vi "Main.vi"() -> ()   [LabVIEW 2015, in "ROOT.lvlib"]
doc: "This template is based off of the Queued Message Handler design pattern and the Queued Message Handler project template that ships with LabVIEW.\n\nThe main difference is that the queue is private to this module and communication between modules is performed via Broadcast and Request events.\n\nRequest events are wrapped in public API methods and are handled in the Event Handling Loop (EHL) of this VI. Any module can register for Broadcast events sent by this module. The EHL generates messages based on user interface actions.\n\nThe Message Handling Loop (MHL) processes messages generated by the EHL, or by other messages. The messages are string values, so new messages can be added easily to the Message Cases case structure in the MHL. Each message cluster can also provide an optional value for Message Data, which is a variant that can be converted to whatever message-specific data is required.\n_____\nBased on Delacor QMH Project Template 4.2.1.64."
uses:
  ROOT.lvlib
  <vilib>/Delacor/Delacor QMH/Libraries/Module Admin_class/Delacor_lib_QMH_Module Admin.lvclass
  Module Data--cluster.ctl
  <vilib>/Delacor/Delacor QMH/Libraries/Message Queue_class/Delacor_lib_QMH_Message Queue.lvclass/Delacor_lib_QMH_Message Queue.ctl
  Stop Argument--cluster.ctl
  <vilib>/Delacor/Delacor QMH/Libraries/Module Admin_class/Delacor_lib_QMH_Module Admin.lvclass/Delacor_lib_QMH_Module Admin.ctl
  <vilib>/Utility/miscctls.llb/LVPointTypeDef.ctl
  <vilib>/Delacor/Delacor QMH/Libraries/Message Queue_class/Delacor_lib_QMH_Enqueue Message (Single).vi
  <vilib>/Delacor/Delacor QMH/Libraries/Module Admin_class/Delacor_lib_QMH_Get External Launch.vi
  <vilib>/Utility/error.llb/Error Cluster From Error Code.vi
  <vilib>/ErrorRing/Error Ring.xnode
  <vilib>/Delacor/Delacor QMH/Libraries/Message Queue_class/Delacor_lib_QMH_Message Queue.lvclass
  Control/Control.lvlib
panel:
  in  "Stop Thermo Chamber":bool
  out "Initialized?":bool
  in  "Starting Temperature":dbl format="%#_13g"
  in  "Start Thermochamber":bool
  out "Hardware Alias":string
  in  "Get Hardware Number":bool
  in  "Simulate MHL Error":bool
  in  "Simulate EHL Error":bool
  out "error out":errorcluster
  in  "Module Admin":refnum<class "Delacor_lib_QMH_Module Admin.lvclass">
  out "Status":string
  # "ROOT Module\n**This module could be used to launch lots of other hardware modules and used to link them to the rest of the application**"
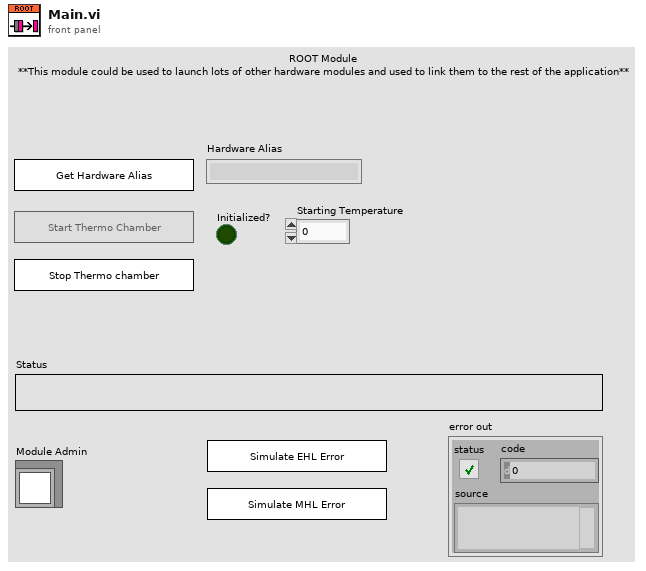
[diagram p1: front panel]
types:
  T1 = typedef "ROOT.lvlib/Request Events--cluster.ctl" = cluster{"Stop Module":refnum<user-event>, "Show Panel":refnum<user-event>, "Hide Panel":refnum<user-event>, "Get Module Execution Status":refnum<user-event>, "Show Diagram":refnum<user-event>}
  T2 = typedef "Control.lvlib/Broadcast Events--cluster.ctl" = cluster{"Module Did Init":refnum<user-event>, "Status Updated":refnum<user-event>, "Error Reported":refnum<user-event>, "Module Did Stop":refnum<user-event>, "Update Module Execution Status":refnum<user-event>, "Thermochamber Started":refnum<user-event>, "Thermochamber Stopped":refnum<user-event>}
  T3 = typedef "ROOT.lvlib/Module Data--cluster.ctl" = cluster{"Status":string}
  T4 = enum8{"Enabled", "Disabled", "Disabled and Grayed Out"}
  T5 = enum32{"invalid lock state", "Not Locked", "Locked (No Password)", "Password-protected"}
  T6 = typedef "ROOT.lvlib/Stop Argument--cluster.ctl" = cluster{"Origin":string, "Exit via Stop Module Req?":bool, "Wait for Module to stop?":bool}
  T7 = typedef "LVPointTypeDef.ctl" = cluster{"Horizontal":i16, "Vertical":i16}
  T8 = enum32{"Invalid", "Standard", "Closed", "Hidden", "Minimized", "Maximized"}
  T9 = typedef "Control.lvlib/Get Hardware Alias (Reply Payload)--cluster.ctl" = cluster{"Hardware Alias":string, "Get Hardware Alias_error":errorcluster}
  T10 = typedef "Control.lvlib/Start Thermochamber (Reply Payload)--cluster.ctl" = cluster{"Initialized?":bool, "Start Thermochamber_error":errorcluster}
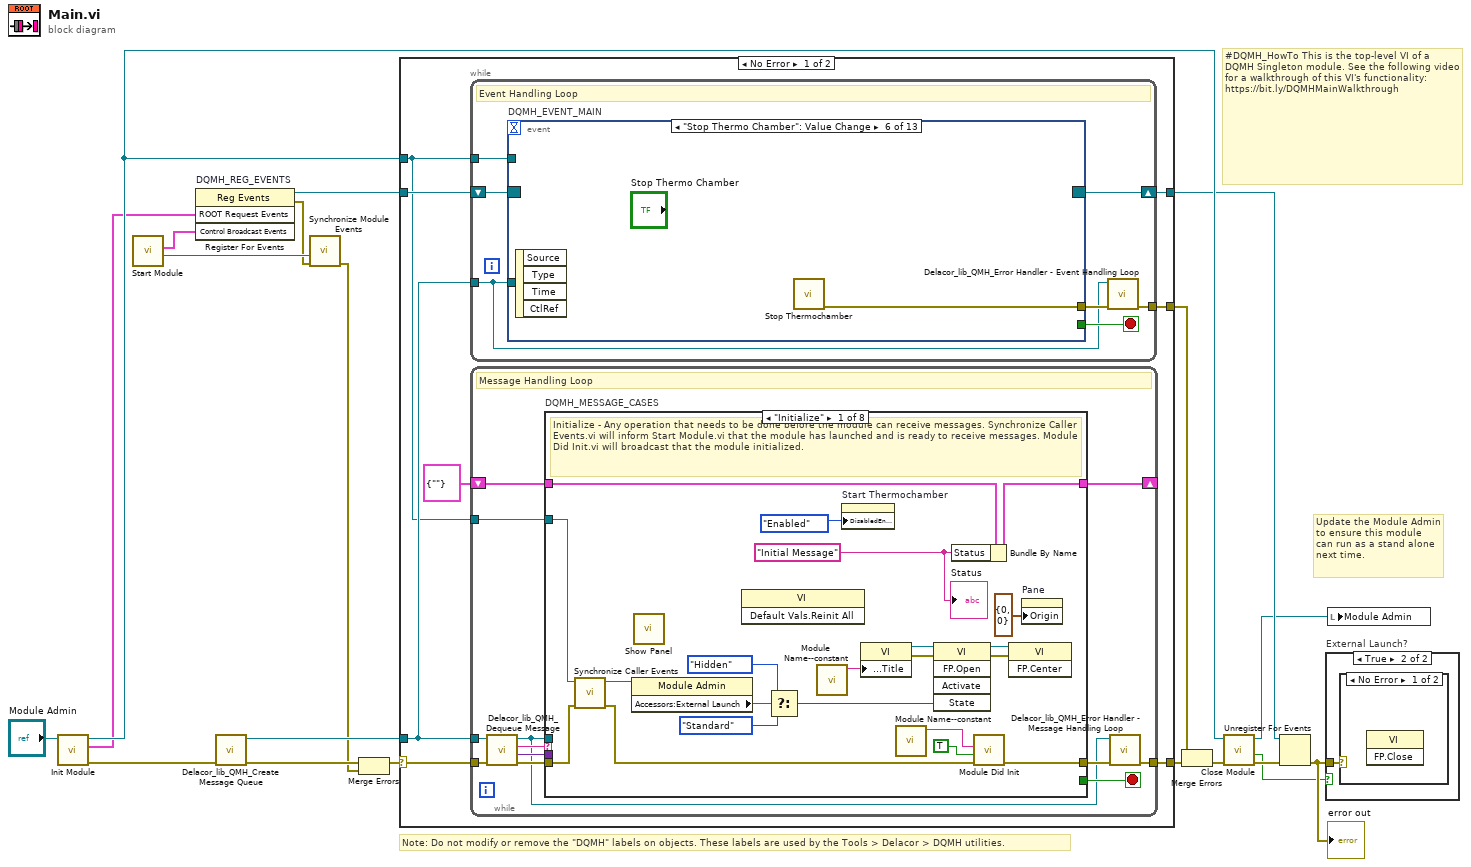
[diagram p0: block diagram]
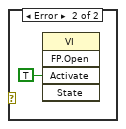
[diagram p3: hidden frame]
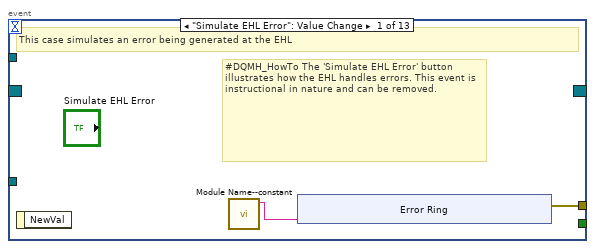
[diagram p4: hidden frame]
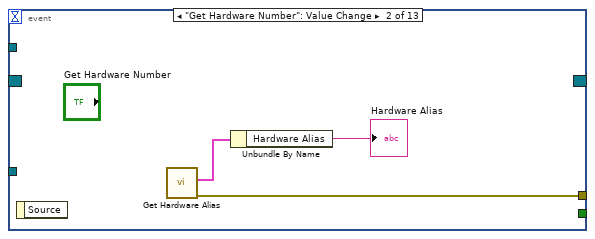
[diagram p5: hidden frame]
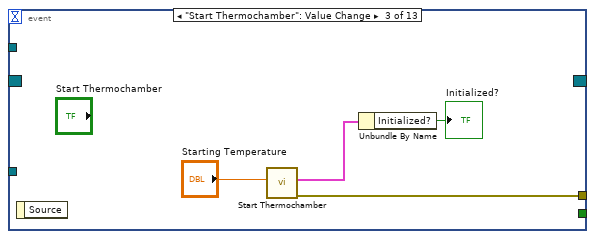
[diagram p6: hidden frame]
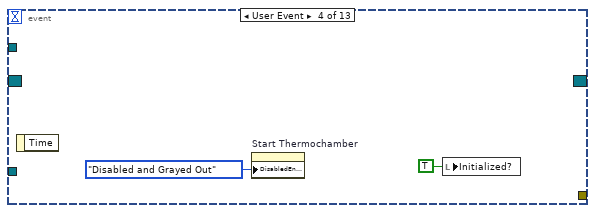
[diagram p7: hidden frame]
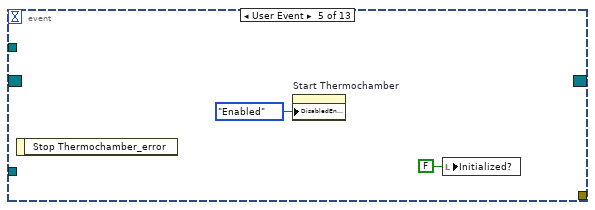
[diagram p8: hidden frame]
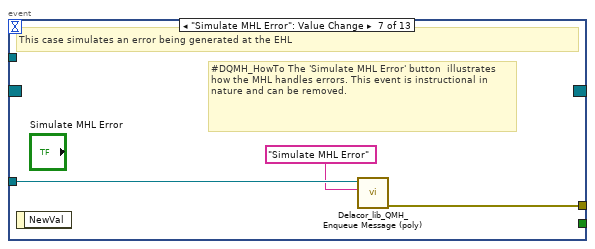
[diagram p9: hidden frame]
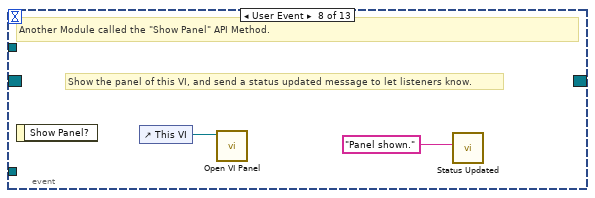
[diagram p10: hidden frame]
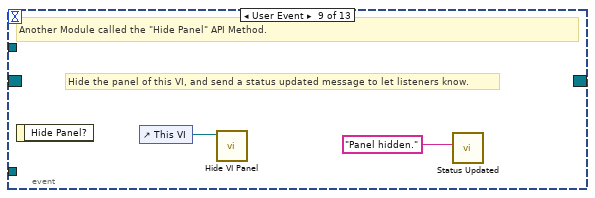
[diagram p11: hidden frame]
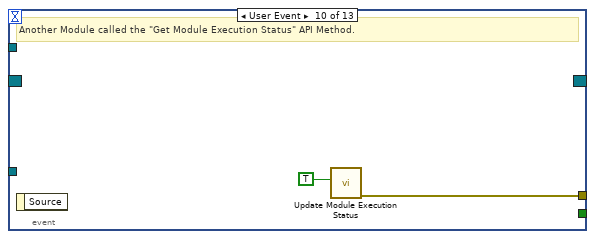
[diagram p12: hidden frame]
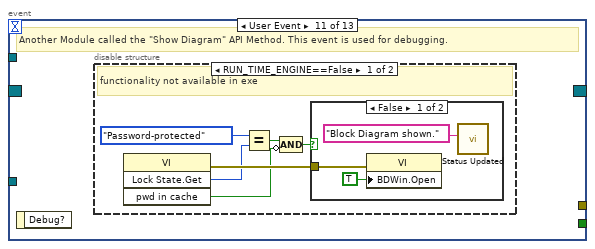
[diagram p13: hidden frame]
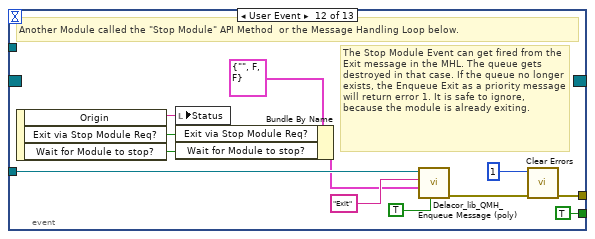
[diagram p16: hidden frame]
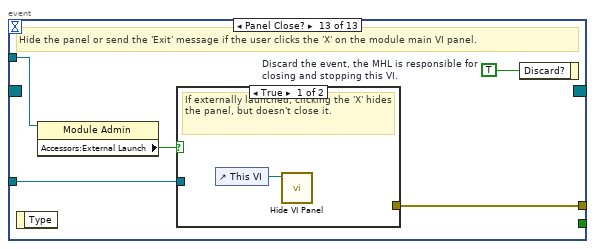
[diagram p17: hidden frame]
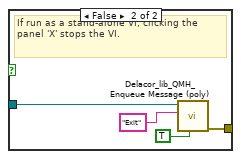
[diagram p18: hidden frame]
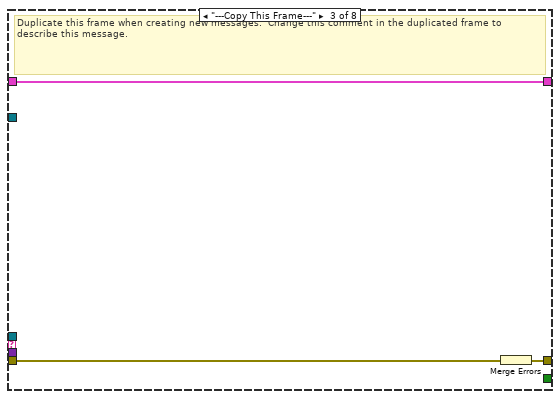
[diagram p20: hidden frame]
diagram:
  # "#DQMH_HowTo This is the top-level VI of a DQMH Singleton module. See the following video for a walkthrough of this VI's functionality: https://bit.ly/DQMHMainWalkthrough"
  # "Note: Do not modify or remove the \"DQMH\" labels on objects. These labels are used by the Tools > Delacor > DQMH utilities."
  # "Update the Module Admin to ensure this module can run as a stand alone next time."
  n1 = call "Init Module.vi"("Singleton Module Admin in"="Module Admin") -> ("error out"=w19:errorcluster, "ROOT Request Events"=w9:T1, "Singleton Module Admin out"=w12:refnum<class "Delacor_lib_QMH_Module Admin.lvclass">)  [unwired: 8 in]
  n2 = call "Start Module.vi"() -> ("Wait for Event Sync?"=w3:bool, "Control Broadcast Events"=w4:T2)  [unwired: 8 in, 2 out]
  n3 = register-events "DQMH_REG_EVENTS"(w9, w4) -> (reference out=w10:refnum<event-registration>, error out=w2:errorcluster)  [unwired: 2 in]
  n4 = call <vilib>:"Delacor_lib_QMH_Create Message Queue.vi"("error in (no error)"=w19) -> ("error out"=w14:errorcluster, "Message Queue"=w8:refnum<class "Delacor_lib_QMH_Message Queue.lvclass">)  [unwired: 9 in]
  n5 = call "Synchronize Module Events.vi"("error in (no error)"=w2, "Wait for Event Sync?"=w3) -> ("error out"=w1:errorcluster)  [unwired: 9 in]
  n6 = Merge Errors(w14, w1) -> (w13:errorcluster)
  n7 = case shown="No Error" w13 {
    selector: w13 -> [w26 w201]
    tunnel: [w28 w201] -> w20
    tunnel: [w25 w198] -> w11
    tunnel: w10 -> [w23 w198]
    tunnel: w8 -> [w22 _]
    tunnel: [w27 _] -> w17
    tunnel: w12 -> [w21 w194]
    frame No Error {
      n8 = while {
        tunnel: w22 -> [w29]
        shift-right: [w32] -> w25
        shift-left: w23 -> [w33]
        tunnel: [w34] -> w27
        tunnel: w21 -> [w30]
        stop <- w31 stop-if-true
        # "Event Handling Loop"
        n9 = event "DQMH_EVENT_MAIN" shown="[5] \"Stop Thermo Chamber\": Value Change" {
          selector: w33 -> [_ _ _ _ _ _ _ _ _ _ _ _ _]
          dyn-events: [_ _ _ _ _ _ _ _ _ _ _ _ _] -> w32
          timeout: _ -> [_ _ _ _ _ _ _ _ _ _ _ _ _]
          tunnel: [_ _ _ _ _ _ _ _ _ _ _ TRUE ("Discard?") _] -> w31
          tunnel: w29 -> [_ _ _ _ _ _ w58 _ _ _ _ w82 w89]
          tunnel: [w37 w47 w51 _ _ w56 w59 _ _ w65 _ w85 w91] -> w35
          tunnel: w30 -> [_ _ _ _ _ _ _ _ _ _ _ _ w88]
          event "Simulate EHL Error": Value Change {
            # "#DQMH_HowTo The 'Simulate EHL Error' button  illustrates how the EHL handles errors. This event is instructional in nature and can be removed."
            # "This case simulates an error being generated at the EHL"
            n10 = event-data() -> ()  [unwired: 1 in, 1 out]
            n11 = call "Module Name--constant.vi"() -> ("Module Name"=w36:string)  [unwired: 11 in]
            n12 = xnode "Error Ring"("parameter 0"=w36) -> ("error out"=w37:errorcluster)
          }
          event "Get Hardware Number": Value Change {
            n13 = event-data() -> ()  [unwired: 1 in, 1 out]
            n14 = call "Get Hardware Alias.vi"() -> ("error out"=w47:errorcluster, "Reply Payload"=w46:T9)  [unwired: 9 in, 1 out]
            n15 = Unbundle By Name(w46) -> ("Hardware Alias"=→"Hardware Alias":string)
          }
          event "Start Thermochamber": Value Change {
            n16 = event-data() -> ()  [unwired: 1 in, 1 out]
            n17 = call "Start Thermochamber.vi"("Initial Starting Temperature"="Starting Temperature") -> ("error out"=w51:errorcluster, "Reply Payload"=w49:T10)  [unwired: 8 in, 1 out]
            n18 = Unbundle By Name(w49) -> ("Initialized?"=→"Initialized?":bool)
          }
          event User Event {
            n19 = event-data() -> ()  [unwired: 1 in, 1 out]
            n20 = property on="Start Thermochamber" class="Bool"("DisabledEnum"=T4."Disabled and Grayed Out" ("Disabled")) -> ()  [unwired: 2 in, 2 out]
            n21 = local write "Initialized?"(TRUE ("Initialized?")) -> ()
          }
          event User Event {
            n22 = event-data() -> ()  [unwired: 1 in, 1 out]
            n23 = property on="Start Thermochamber" class="Bool"("DisabledEnum"=T4."Enabled" ("Disabled")) -> ()  [unwired: 2 in, 2 out]
            n24 = local write "Initialized?"(FALSE ("Initialized?")) -> ()
          }
          event "Stop Thermo Chamber": Value Change {
            n25 = event-data() -> ()  [unwired: 1 in, 4 out]
            n26 = call "Stop Thermochamber.vi"() -> ("error out"=w56:errorcluster)  [unwired: 9 in, 2 out]
          }
          event "Simulate MHL Error": Value Change {
            # "#DQMH_HowTo The 'Simulate MHL Error' button  illustrates how the MHL handles errors. This event is instructional in nature and can be removed."
            # "This case simulates an error being generated at the EHL"
            n27 = event-data() -> ()  [unwired: 1 in, 1 out]
            n28 = call-poly <vilib>:"Delacor_lib_QMH_Enqueue Message (poly).vi"("Message"="Simulate MHL Error", "Message Queue in"=w58) -> ("error out"=w59:errorcluster)  [unwired: 8 in, 1 out]
          }
          event User Event {
            # "Show the panel of this VI, and send a status updated message to let listeners know."
            # "Another Module called the \"Show Panel\" API Method."
            n29 = event-data() -> ()  [unwired: 1 in, 1 out]
            n30 = control-ref of="This VI"() -> (w61:refnum<vi>)
            n31 = call "Open VI Panel.vi"("VI"=w61) -> ()  [unwired: 10 in, 1 out]
            n32 = call "Status Updated.vi"("Status"="Panel shown." ("format string")) -> ()  [unwired: 10 in, 1 out]
          }
          event User Event {
            # "Hide the panel of this VI, and send a status updated message to let listeners know."
            # "Another Module called the \"Hide Panel\" API Method."
            n33 = event-data() -> ()  [unwired: 1 in, 1 out]
            n34 = control-ref of="This VI"() -> (w63:refnum<vi>)
            n35 = call "Hide VI Panel.vi"("VI"=w63) -> ()  [unwired: 10 in, 1 out]
            n36 = call "Status Updated.vi"("Status"="Panel hidden." ("format string")) -> ()  [unwired: 10 in, 1 out]
          }
          event User Event {
            # "Another Module called the \"Get Module Execution Status\" API Method."
            n37 = event-data() -> ()  [unwired: 1 in, 1 out]
            n38 = call "Update Module Execution Status.vi"("Running?"=TRUE) -> ("error out"=w65:errorcluster)  [unwired: 10 in]
          }
          event User Event {
            # "Another Module called the \"Show Diagram\" API Method. This event is used for debugging."
            n39 = event-data() -> ()  [unwired: 1 in, 1 out]
            n40 = disable-structure shown="RUN_TIME_ENGINE==False" {
              frame condition #0 (active) {
                # "functionality not available in exe"
                n41 = invoke class="VI" method="Lock State.Get"() -> (error out=w71:errorcluster, "Get Lock State"=w70:T5, "pwd in cache"=w67:bool)  [unwired: 4 in, 1 out]
                n42 = Equal?(x=T5."Password-protected", y=w70) -> (x = y?=w68:bool)
                n43 = Compound Arithmetic op=AND(w68, invert w67) -> (w66:bool)
                n44 = case shown="False" w66 {
                  tunnel: w71 -> [w74 _]
                  frame False {
                    n45 = property class="VI"(error in=w74, "BDWin.Open"=TRUE ("Block Diagram Window:Open")) -> ()  [unwired: 1 in, 2 out]
                    n46 = call "Status Updated.vi"("Status"="Block Diagram shown." ("format string")) -> ()  [unwired: 10 in, 1 out]
                  }
                  frame True {
                    # "Password-protected VI, and the password is not in the cache. Do not show the diagram."
                  }
                }
              }
              frame condition #1 {
              }
            }
          }
          event User Event {
            # "The Stop Module Event can get fired from the Exit message in the MHL. The queue gets destroyed in that case. If the queue no longer exists, the Enqueue Exit as a priority message will return error 1. It is safe to ignore, because the module is already exiting."
            # "Another Module called the \"Stop Module\" API Method  or the Message Handling Loop below."
            n47 = event-data() -> ("Origin"=w81:string, "Exit via Stop Module Req?"=w77:bool, "Wait for Module to stop?"=w76:bool)  [unwired: 1 in]
            n48 = local write "Status"(w81) -> ()
            n49 = Bundle By Name(cluster=T6 {"Origin"="", "Exit via Stop Module Req?"=FALSE, "Wait for Module to stop?"=FALSE} ("Stop Argument"), "Exit via Stop Module Req?"=w77, "Wait for Module to stop?"=w76) -> (w75:T6)
            n50 = call-poly <vilib>:"Delacor_lib_QMH_Enqueue Message (poly).vi"("Priority Message? (F)"=TRUE, "Message Data"=w75, "Message"="Exit", "Message Queue in"=w82) -> ("error out"=w86:errorcluster)  [unwired: 6 in, 1 out]
            n51 = call <vilib>:"Clear Errors.vi"("error in (no error)"=w86, "specific error code to clear (0: all)"=1) -> ("error out"=w85:errorcluster)  [unwired: 4 in, 1 out]
          }
          event Panel Close? {
            w90 = TRUE  # Discard the event, the MHL is responsible for closing and stopping this VI.
            # "Hide the panel or send the 'Exit' message if the user clicks the 'X' on the module main VI panel."
            n52 = event-data() -> ()  [unwired: 1 in, 1 out]
            n53 = property class="Module Admin"(reference=w88) -> ("Accessors:External Launch"=w87:bool)  [unwired: 1 in, 2 out]
            n54 = case shown="True" w87 {
              tunnel: w89 -> [_ w95]
              tunnel: [_ w96] -> w91
              frame True {
                # "If externally launched, clicking the 'X' hides the panel, but doesn't close it."
                n55 = control-ref of="This VI"() -> (w92:refnum<vi>)
                n56 = call "Hide VI Panel.vi"("VI"=w92) -> ()  [unwired: 10 in, 1 out]
              }
              frame False {
                # "If run as a stand-alone VI, clicking the panel 'X' stops the VI."
                n57 = call-poly <vilib>:"Delacor_lib_QMH_Enqueue Message (poly).vi"("Priority Message? (F)"=TRUE, "Message"="Exit", "Message Queue in"=w95) -> ("error out"=w96:errorcluster)  [unwired: 7 in, 1 out]
              }
            }
            n58 = event-data("Discard?"=w90) -> ()  [unwired: 1 in, 1 out]
          }
        }
        n59 = call-dynamic "Delacor_lib_QMH_Error Handler - Event Handling Loop.vi"("error in (no error)"=w35, "Message Queue in"=w29) -> ("dup error in"=w34:errorcluster)  [unwired: 8 in, 1 out]
      }
      n60 = while {
        tunnel: w22 -> [w99]
        shift-right: [w103] -> _
        shift-left: T3 {"Status"=""} ("Data Cluster") -> [w104]
        tunnel: w26 -> [w107]
        tunnel: [w105] -> w28
        tunnel: w21 -> [w97]
        stop <- w102 stop-if-true
        # "Message Handling Loop"
        n61 = call-dynamic "Delacor_lib_QMH_Dequeue Message.vi"("error in (no error)"=w107, "Message Queue in"=w99) -> ("error out"=w106:errorcluster, "Message Data"=w100:variant, "Message"=w101:string, "Message Queue out"=w98:refnum<class "Delacor_lib_QMH_Message Queue.lvclass">)  [unwired: 6 in]
        n62 = case "DQMH_MESSAGE_CASES" shown="\"Initialize\"" w101 {
          selector: w101 -> [_ _ _ _ _ _ _ w181]
          tunnel: w98 -> [_ _ _ _ _ w151 w173 _]
          tunnel: w106 -> [w127 w131 w134 w136 w141 w158 w179 w183]
          tunnel: [w125 w131 w133 w136 w140 w154 w176 w184] -> w108
          tunnel: w104 -> [w116 w130 w132 w135 w138 w153 w172 w182]
          tunnel: [w115 w130 w132 w135 w138 w153 w172 w182] -> w103
          tunnel: [_ _ _ _ _ _ w171 _] -> w102
          tunnel: w100 -> [_ _ _ _ _ w152 w170 _]
          tunnel: w97 -> [w117 _ _ _ _ w150 w165 _]
          frame "Initialize" {
            w110 = "Initial Message" ("Initial Message")
            # "Initialize - Any operation that needs to be done before the module can receive messages. Synchronize Caller Events.vi will inform Start Module.vi that the module has launched and is ready to receive messages. Module Did Init.vi will broadcast that the module initialized."
            n63 = call "Synchronize Caller Events.vi"("error in (no error)"=w127, "Singleton Module Admin in"=w117) -> ("error out"=w126:errorcluster, "Singleton Module Admin out"=w112:refnum<class "Delacor_lib_QMH_Module Admin.lvclass">)  [unwired: 8 in]
            n64 = property class="Module Admin"(reference=w112) -> ("Accessors:External Launch"=w121:bool)  [unwired: 1 in, 2 out]
            n65 = call "Show Panel.vi"() -> ()  [unwired: 11 in, 1 out]
            n66 = invoke class="VI" method="Default Vals.Reinit All"() -> ()  [unwired: 3 in, 3 out]
            n67 = Select(t=T8."Hidden" ("State"), s=w121, f=T8."Standard" ("State")) -> (s? t:f=w118:T8)
            n68 = call "Module Name--constant.vi"() -> ("Module Name"=w124:string)  [unwired: 11 in]
            n69 = property on="Start Thermochamber" class="Bool"("DisabledEnum"=T4."Enabled" ("Disabled")) -> ()  [unwired: 2 in, 2 out]
            n70 = property class="VI"("Front Panel.Title"=w124) -> (reference out=w123:refnum<vi>, error out=w129:errorcluster)  [unwired: 2 in]
            n71 = call "Module Name--constant.vi"() -> ("Module Name"=w113:string)  [unwired: 11 in]
            n72 = invoke class="VI" method="FP.Open"(reference=w123, error in=w129, "State"=w118) -> (reference out=w122:refnum<vi>, error out=w128:errorcluster)  [unwired: 2 in, 3 out]
            n73 = Bundle By Name(cluster=w116, "Status"=w110) -> (w115:T3)
            n74 = call "Module Did Init.vi"("error in (no error)"=w126, "Initialized?"=TRUE, "Origin"=w113) -> ("error out"=w125:errorcluster)  [unwired: 8 in]
            n75 = invoke class="VI" method="FP.Center"(reference=w122, error in=w128) -> ()  [unwired: 1 in, 3 out]
            n76 = property on="Pane" class="Pane"("Origin"=T7 {"Horizontal"=0, "Vertical"=0}) -> ()  [unwired: 2 in, 2 out]
            "Status" <- w110
          }
          frame "--- Module Specific ---" {
            # "Separator -- The following cases handle messages specific to this Module."
          }
          frame "---Copy This Frame---" {
            # "Duplicate this frame when creating new messages.  Change this comment in the duplicated frame to describe this message."
            n77 = Merge Errors(w134) -> (w133:errorcluster)
          }
          frame "--- Exit and Error Handling---" {
            # "Separator - The following cases handle errors and exit messages."
          }
          frame "Simulate MHL Error" {
            # "#DQMH_HowTo The 'Simulate MHL Error' button  illustrates how the MHL handles errors. This event is instructional in nature and can be removed."
            # "Simulate an error occurring at the MHL"
            n78 = call "Module Name--constant.vi"() -> ("Module Name"=w137:string)  [unwired: 11 in]
            n79 = xnode "Error Ring"("parameter 0"=w137) -> ("error out"=w139:errorcluster)
            n80 = Merge Errors(w141, w139) -> (w140:errorcluster)
          }
          frame "Error" {
            # "#CodeRecommended - If you ever change the name of this \"Error\" message, you'll need to update the name in the Check Loop Error.vi as well."
            # "#CodeRecommended - If the module is running in standalone mode (External Launch = FALSE), this code will pop up an error dialog and call the 'Exit' message if an error occurs. Add more fine-grained error handling here."
            # "Error - Check the error message data and respond accordingly. This message is sent by the \"Error Handler\" VIs at the end of each loop in this application."
            n81 = property class="Module Admin"(reference=w150) -> ("Accessors:External Launch"=w149:bool)  [unwired: 1 in, 2 out]
            n82 = Variant To Data(error in=w158, type=errorcluster {"status"=FALSE, "code"=0, "source"=""} ("error constant"), Variant=w152) -> (data=w159:errorcluster, error out=w156:errorcluster)
            n83 = call "Error Reported.vi"("Error"=w159) -> ()  [unwired: 10 in, 1 out]
            n84 = case shown="False" w149 {
              tunnel: [w164 _] -> w155
              tunnel: w151 -> [w162 _]
              tunnel: w159 -> [w163 _]
              frame False {
                # "If the module is running standalone, then pop up an error dialog and call the \"Exit\" message."
                n85 = call <vilib>:"Simple Error Handler.vi"("error in (no error)"=w163) -> ()  [unwired: 4 in, 5 out]
                n86 = call-poly <vilib>:"Delacor_lib_QMH_Enqueue Message (poly).vi"("Priority Message? (F)"=TRUE, "Message"="Exit", "Message Queue in"=w162) -> ("error out"=w164:errorcluster)  [unwired: 7 in, 1 out]
              }
              frame True {
                # "If the module was launched externally, calling the Error Reported broadcast VI is the only action performed by the \"Error\" message. The module's caller can then process the error appropriately."
              }
            }
            n87 = Merge Errors(w156, w155) -> (w154:errorcluster)
            n88 = local write "error out"(w154) -> ()
          }
          frame "Exit" {
            w169 = 91  # 91: not all Exit messages will have an argument
            w171 = TRUE  # Stop the VI
            # "Release the message queue reference"
            # "#CodeNeeded - Add any required cleanup code here"
            # "Exit - Exit the application."
            n89 = Variant To Data(error in=w179, type=T6 {"Origin"="", "Exit via Stop Module Req?"=FALSE, "Wait for Module to stop?"=FALSE} ("Stop Argument"), Variant=w170) -> (data=w167:T6, error out=w175:errorcluster)
            n90 = call <vilib>:"Clear Errors.vi"("error in (no error)"=w175, "specific error code to clear (0: all)"=w169) -> ("error out"=w178:errorcluster)  [unwired: 4 in, 1 out]
            n91 = control-ref of="This VI"() -> (w166:refnum<vi>)
            n92 = call-dynamic "Delacor_lib_QMH_Release Message Queue.vi"("error in (no error)"=w178, "Message Queue"=w173) -> ("error out"=w177:errorcluster)  [unwired: 9 in]
            n93 = call "Handle Exit.vi"("Stop Argument"=w167, "Admin in"=w165, "VI reference"=w166) -> ("error out"=w174:errorcluster)  [unwired: 7 in, 1 out]
            n94 = Merge Errors(w177, w174) -> (w176:errorcluster)
            n95 = call "Stop Module.vi"() -> ()  [unwired: 11 in, 1 out]
          }
          frame Default {
            # "'Default' case only runs if there is a message that isn't defined in any of the other cases.  Output a programming error."
            n96 = call "Module Name--constant.vi"() -> ("Module Name"=w180:string)  [unwired: 11 in]
            n97 = xnode "Error Ring"("parameter 0"=w181, "parameter 1"=w180) -> ("error out"=w185:errorcluster)
            n98 = Merge Errors(w183, w185) -> (w184:errorcluster)
          }
        }
        n99 = call-dynamic "Delacor_lib_QMH_Error Handler - Message Handling Loop.vi"("error in (no error)"=w108, "Message Queue in"=w98) -> ("dup error in"=w105:errorcluster)  [unwired: 8 in, 1 out]
      }
    }
    frame Error {
      # "Synchronize Caller Events.vi will inform Start Module.vi that the module has launched and will let the code calling Start Module.vi register for broadcasts and would permit the caller receive the broadcast that an error occurred at launch time."
      n100 = call "Synchronize Caller Events.vi"("Singleton Module Admin in"=w194) -> ("error out"=w199:errorcluster)  [unwired: 9 in, 1 out]
      n101 = call "Module Name--constant.vi"() -> ("Module Name"=w197:string)  [unwired: 11 in]
      n102 = Format Into String(format string="An error occurred during initialization. %s is no longer running.", w197) -> (resulting string=w195:string)  [unwired: 2 in, 1 out]
      n103 = Merge Errors(w201, w199) -> (w200:errorcluster)
      n104 = call "Error Reported.vi"("Additional Information"=w195, "Error"=w200) -> ()  [unwired: 9 in, 1 out]
    }
  }
  n105 = Merge Errors(w17, w20) -> (w16:errorcluster)
  n106 = call "Close Module.vi"("error in (no error)"=w16, "Module Admin in"=w12) -> ("error out"=w18:errorcluster, "External Launch"=w5:bool, "Module Admin out"=w6:refnum<class "Delacor_lib_QMH_Module Admin.lvclass">)  [unwired: 7 in]
  n107 = Unregister For Events(event registration refnum=w11, error in=w18) -> (error out=w15:errorcluster)
  "error out" <- w15
  n108 = case "External Launch?" shown="True" w5 {
    tunnel: w15 -> [_ w202]
    frame False {
    }
    frame True {
      n109 = case shown="No Error" w202 {
        frame No Error {
          n110 = invoke class="VI" method="FP.Close"() -> ()  [unwired: 3 in, 3 out]
        }
        frame Error {
          n111 = invoke class="VI" method="FP.Open"("Activate"=TRUE ("Activate?")) -> ()  [unwired: 4 in, 5 out]
        }
      }
    }
  }
  n112 = local write "Module Admin"(w6) -> ()
